vi "setRoot.vi"(8 "error in (no error)":errorcluster, 10 "Root":refnum<data-value>, 11 "LinkedList in":refnum<class "LinkedList.lvclass">) -> (0 "error out":errorcluster, 3 "LinkedList out":refnum<class "LinkedList.lvclass">)   [LabVIEW 2009, in "LinkedList.lvclass"]
doc: "Sets the frontmost node of the linked list, referred to as the root node."
uses:
  LinkedList.lvclass
  LLNode/LLNode.lvclass
  LinkedList.lvclass/LinkedList.ctl
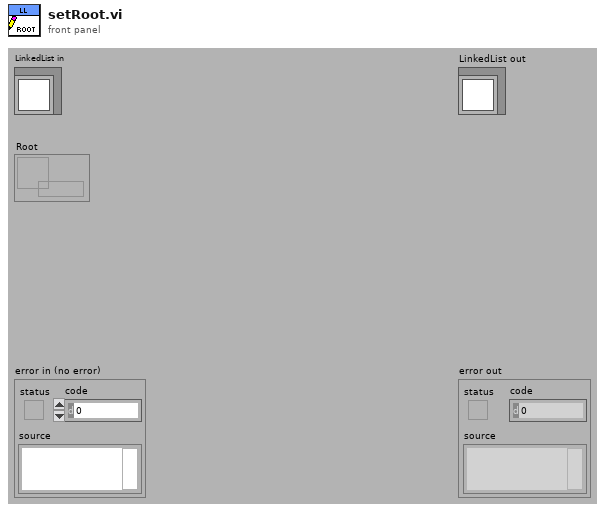
[diagram p1: front panel]
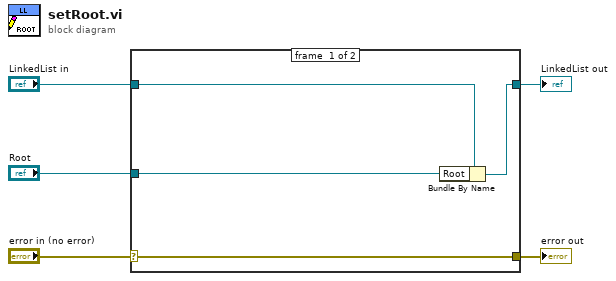
[diagram p0: block diagram]
diagram:
  n1 = case shown="No Error" "error in (no error)" {
    selector: "error in (no error)" -> [w9 w10]
    tunnel: [w9 w10] -> w4
    tunnel: [w7 w11] -> w2
    tunnel: "LinkedList in" -> [w8 w11]
    tunnel: "Root" -> [w6 _]
    frame #0 {
      n2 = Bundle By Name(cluster=w8, "Root"=w6) -> (w7:refnum<class "LinkedList.lvclass">)
    }
    frame #1 {
    }
  }
  "error out" <- w4
  "LinkedList out" <- w2
